vi "Drive Forward Auto.vi"(7 "Mecanum":bool, 8 "error in (no error)":errorcluster, 9 "Time (s)":dbl, 10 "Forward Speed":dbl, 11 "refnum name":string="RobotDrive") -> (0 "error out":errorcluster)   [LabVIEW 2014]
doc: "A basic auto that drives forward and stops."
uses:
  <vilib>/Rock Robotics/WPI/RobotDrive/WPI_RobotDriveGetSetRefNum.vi
  <vilib>/Rock Robotics/WPI/RobotDrive/WPI_RobotDriveArcadeDrive_Standard(NoSaturation).vi
  <vilib>/Rock Robotics/WPI/RobotDrive/WPI_RobotDriveMecanumDrive_Cartesian.vi
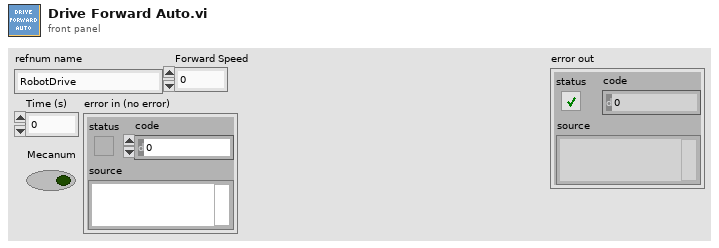
[diagram p1: front panel]
types:
  T1 = typedef "WPI_RobotDriveDevRef.ctl" = cluster{"DevStatus":errorcluster, "Motors[]":T2[], "Square Inputs":bool, "Max Output":dbl}
  T2 = typedef "WPI_MotorControlDeviceRef.ctl" = cluster{"DeviceStatus":errorcluster, "Type":T3, "PWM":cluster{"Controller":T4, "PWM Channel":T5, "DeadBand":T6}, "CAN":cluster{"Device Number":u8, "Control Mode":T7, "Semaphore":T8, "Max Vout":dbl, "TalonSRX Control Mode":T9}, "Invert":bool, "TransformRef":T10, "InvTransformRef":T10}
  T3 = typedef "WPI_MotorControlType.ctl" = enum16{"PWM", "CAN", "CANTalonSRX"}
  T4 = typedef "FPGA_TypedefDigitalModule.ctl" = enum16{"Controller 1"}
  T5 = typedef "FPGA_DIOPWMChannel.ctl" = enum8{"PWM 0", "PWM 1", "PWM 2", "PWM 3", "PWM 4", "PWM 5", "PWM 6", "PWM 7", "PWM 8", "PWM 9", "PWM MXP 0", "PWM MXP 1", "PWM MXP 2", "PWM MXP 3", "PWM MXP 4", "PWM MXP 5", "PWM MXP 6", "PWM MXP 7", "PWM MXP 8", "PWM MXP 9", "Invalid"}
  T6 = typedef "WPI_PWMDeadband.ctl" = cluster{"Name":string, "maxPositivePwm":i32, "minPositivePwm":i32, "centerPwm":i32, "maxNegativePwm":i32, "minNegativePwm":i32, "angularRange":u16}
  T7 = typedef "WPI_CANJaguar_ControlMode.ctl" = enum8{"Percent VBus", "Current", "Speed", "Position", "Voltage"}
  T8 = typedef "Semaphore RefNum" = refnum<k1>
  T9 = typedef "WPI_CANTalonSRX_APIControlMode.ctl" = enum8{"Percent VBus", "Speed", "Position", "Slave", "Unchanged / Invalid"}
  T10 = typedef "WPI_PWMTransform_ConPane.ctl" = refnum<vi>
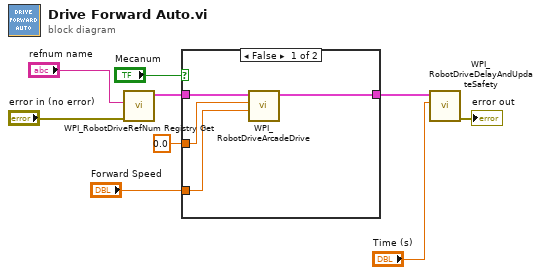
[diagram p0: block diagram]
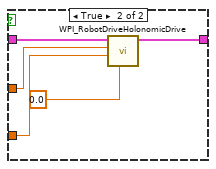
[diagram p2: hidden frame]
diagram:
  n1 = call <vilib>:"WPI_RobotDriveRefNum Registry Get.vi"("error in (no error)"="error in (no error)", "refnum name"="refnum name") -> ("RobotDriveDevRef"=w8:T1)  [unwired: 9 out]
  n2 = case shown="False" "Mecanum" {
    tunnel: [w12 w18] -> w9
    tunnel: w8 -> [w13 w17]
    tunnel: 0.0 ("X axis value") -> [w10 w15]
    tunnel: "Forward Speed" -> [w11 w14]
    frame False {
      n3 = call-poly <vilib>:"WPI_RobotDriveArcadeDrive.vi"("Y axis value"=w11, "X axis value"=w10, "RobotDriveDevRef"=w13) -> ("RobotDriveDevRef"=w12:T1)  [unwired: 6 in, 2 out]
    }
    frame True {
      n4 = call-poly <vilib>:"WPI_RobotDriveHolonomicDrive.vi"("Rotation"=0.0, "Y"=w14, "X"=w15, "RobotDriveDevRef"=w17) -> ("RobotDriveDevRef"=w18:T1)  [unwired: 5 in, 2 out]
    }
  }
  n5 = call <vilib>:"WPI_RobotDriveDelayAndUpdateSafety.vi"("Delay (s)"="Time (s)", "RobotDriveDevRef"=w9) -> ("error out"=→"error out":errorcluster)  [unwired: 8 in, 1 out]
